vi "Get All Nodes of Name.vi"(8 "error in (no error)":errorcluster, 10 "Node Name":string, 11 "Project XML Editor in":refnum<class "Project XML Editor.lvclass">) -> (0 "error out":errorcluster, 2 "Nodes Array out":refnum<k20>[](array[refnum]), 3 "Project XML Editor out":refnum<class "Project XML Editor.lvclass">)   [LabVIEW 2019, in "LVLIBP CD XML Updater.lvlib" / "Project XML Editor.lvclass"]
uses:
  Project XML Editor.lvclass
  Project XML Editor.lvclass/Project XML Editor.ctl
  <resource>/objmgr/DOMUserDefRef.rc
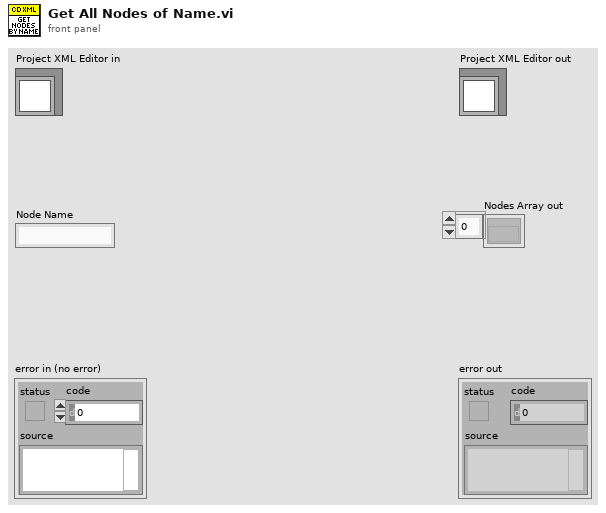
[diagram p1: front panel]
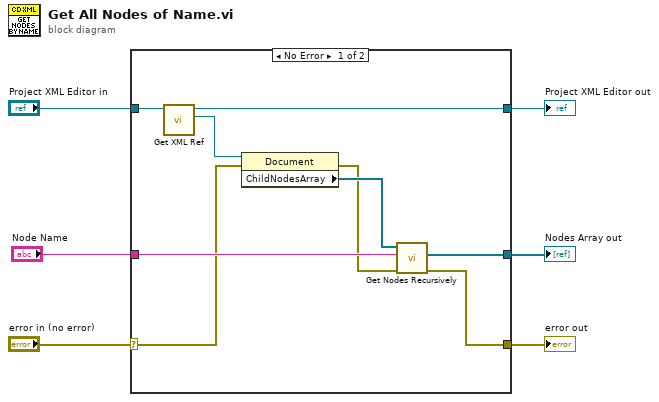
[diagram p0: block diagram]
diagram:
  n1 = case shown="No Error" "error in (no error)" {
    selector: "error in (no error)" -> [w9 w17]
    tunnel: [w10 w17] -> w5
    tunnel: [w13 w16] -> w3
    tunnel: "Project XML Editor in" -> [w14 w16]
    tunnel: "Node Name" -> [w12 _]
    tunnel: [w7 _] -> w1
    frame No Error {
      n2 = call "Get XML Ref.vi"("Project XML Editor in"=w14) -> ("XML Ref"=w15:refnum<k20>, "Project XML Editor out"=w13:refnum<class "Project XML Editor.lvclass">)  [unwired: 9 in]
      n3 = property class="Document"(reference=w15, error in=w9) -> (error out=w8:errorcluster, "ChildNodesArray"=w11:refnum<k20>[])  [unwired: 1 out]
      n4 = call "Get Nodes Recursively.vi"("error in (no error)"=w8, "Node Name"=w12, "Nodes Array in"=w11) -> ("error out"=w10:errorcluster, "Nodes Array out"=w7:refnum<k20>[])  [unwired: 7 in]
    }
    frame Error {
    }
  }
  "error out" <- w5
  "Project XML Editor out" <- w3
  "Nodes Array out" <- w1
